vi "ReadTrajectory_CSV_FIle_WriteGlobal_Example.vi"   [LabVIEW 2019]
uses:
  SubVI/read_csv_StoreTrajectory_GlobalVariable.vi
panel:
  # "Read Trajectory CSV File and \nWrite to Global Variable"
  # "See block diagram"
types:
  T1 = typedef "Trajectory_Library.lvlib/TRAJECTORY.ctl" = cluster{"TotalTImeSecs":dbl, "States":T2[]}
  T2 = typedef "Trajectory_Library.lvlib/TRAJ_STATE.ctl" = cluster{"TimeSeconds":dbl, "Velocity":dbl, "Acceleration":dbl, "POSE":T3, "Curvature":dbl}
  T3 = typedef "Trajectory_Library.lvlib/POSE2D.ctl" = cluster{"TRANSLATION":T4, "ROTATION":T5}
  T4 = typedef "Trajectory_Library.lvlib/TRANSLATION2D.ctl" = cluster{"X":dbl, "Y":dbl}
  T5 = typedef "Trajectory_Library.lvlib/ROTATION2D.ctl" = cluster{"VALUE":dbl, "COS":dbl, "SIN":dbl}
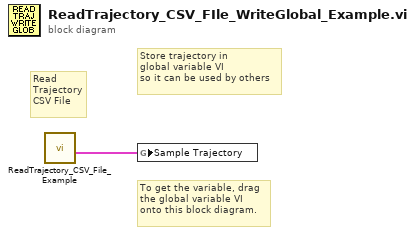
[diagram p0: block diagram]
diagram:
  # "To get the variable, drag\nthe global variable VI\nonto this block diagram."
  # "Read\nTrajectory\nCSV File"
  # "Store trajectory in\nglobal variable VI\nso it can be used by others"
  n1 = call "ReadTrajectory_CSV_File_Example.vi"() -> ("outTRAJECTORY"=w1:T1)  [unwired: 8 in, 3 out]
  n2 = global write "read_csv_StoreTrajectory_GlobalVariable.vi" "Sample Trajectory"(w1) -> ()
